vi "Funktionen Schalten Compact LP Paccar.vi"(8 "Fehler (Eingang)":errorcluster) -> (0 "Fehler (Ausgang)":errorcluster, 2 "Zustand":T1)   [LabVIEW 2020, in "Allgemein.lvlib"]
uses:
  Allgemein.lvlib
  Aktionen FGV Dichtheitstest.ctl
  FGV Zustaende Aktionen.ctl
  Verwaltung/Verwaltung - cRIO.lvlib
  Verwaltung/FGV OUT Aktionen.ctl
  Regler/Regler.lvlib
  Regler/FGV Daten Regler Aktionen.ctl
  Aktion FGV Messbetrieb.ctl
  Funktionstasten/Zustaende.ctl
  Funktionstasten/Funktionstasten.lvlib
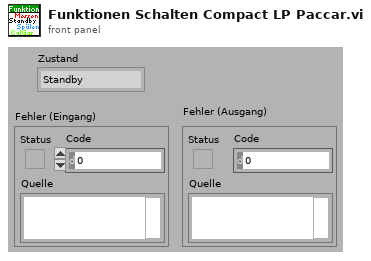
[diagram p1: front panel]
types:
  T1 = typedef "Funktionstasten.lvlib/Zustaende.ctl" = enum16{"Standby", "Pause", "Eco", "Messen", "Kalibrieren", "Spülen Filter", "Spülen Leitung", "Umgebungsluft", "0-Gas", "Cal-Gas", "CG zu PNS", "-------------", "Init 1", "Init 2", "Init 3", "Init 4", "Messen vorbereiten", "Messen durchführen", "Exit"}
  T2 = typedef "Allgemein.lvlib/Aktion FGV Messbetrieb.ctl" = enum16{"lesen", "schreiben"}
  T3 = typedef "Regler.lvlib/FGV Daten Regler Aktionen.ctl" = enum16{"lesen", "Out%", "Heizung EIN"}
  T4 = typedef "Verwaltung - cRIO.lvlib/FGV OUT Aktionen.ctl" = enum16{"lesen", "ANA OUT", "DO 0-31", "DO 32-47"}
  T5 = typedef "Allgemein.lvlib/FGV Zustaende Aktionen.ctl" = enum16{"lesen", "Zustand PC", "Zustand cRIO", "Bildnummer", "Samplepoint", "Sysloglevel"}
  T6 = typedef "Allgemein.lvlib/Aktionen FGV Dichtheitstest.ctl" = enum16{"lesen", "schreiben"}
  T7 = typedef "EPA 1065.lvlib/Dichtheitstest 1065-345.lvlib/Aktion Leak check durchfuehren.ctl" = enum16{"initialisieren", "Unterdruck erzeugen", "Ventile schließen", "Warten", "Auswertung", "fertig", "PDF erstellen"}
  T8 = typedef "Erweiterte Konfig.lvlib/Aktionen Dichtheitstest.ctl" = enum16{"Initialisieren", "Unterdruck aufbauen", "Prop schließen", "Warten", "Auswertung", "Fertig"}
  T9 = cluster{"-23Y1 (CG1)":bool, "-23Y2 (CG2)":bool, "-23Y3 (CG3-10)":bool, "-23Y4 (N2)":bool, "-23Y5":bool, "-27Y2":bool, "-20Y5":bool, "-20Y6":bool, "-20Y7":bool, "-20Y8":bool, "-27Y3":bool, "-27Y4":bool, "Pumpe":bool, "Kondensat":bool, "-22Y3":bool, "-20Y2":bool, "-21Y3":bool, "Absaugung":bool, "-21Y5":bool, "CG zu Entnahme":bool, "-20Y2 (CG3)":bool, "-20Y3 (CG4)":bool, "-20Y4 (CG5)":bool, "-20Y5 (CG6)":bool, "-20Y6 (CG7)":bool, "-20Y7 (CG8)":bool, "-20Y8 (CG9)":bool, "-21Y1 (CG10)":bool}
  T10 = typedef "Verwaltung - cRIO.lvlib/Digital Ausgaenge 32-63.ctl" = cluster{"O32: Messgaspumpe EIN":bool, "O33: (Umgebungsluftpumpe)":bool, "O34: (Kondensatpumpe GK)":bool, "O35: Klima/Lüfter EIN":bool, "O36: Versorgung Heizungen":bool, "O37: Versorgung Heizungen":bool, "O38: (Gaskühler EIN (Freigabe))":bool, "O39: Störung FAS LP":bool, "O40: (Heizung Filterblock)":bool, "O41: Heizung HL zu FT-IR":bool, "O42: Heizung HL Extern SP1":bool, "O43: Heizung HL Extern SP2":bool, "O44: Heizung Reserve":bool, "O45: Heizung Reserve":bool, "O46: Statusbeleuchtung grün":bool, "O47: Statusbeleuchtung rot":bool}
  T11 = typedef "Verwaltung - cRIO.lvlib/Digital Ausgaenge 0-31.ctl" = cluster{"O0: Druckluft Versorgung":bool, "O1: CG 3 (FB Eingang 1)":bool, "O2: CG 4 (Kühlung FT-IR EIN)":bool, "O3: CG 5 (FB Bypass)":bool, "O4: CG 6 (FB CalGas)":bool, "O5: CG 7 (FB spülen/UL)":bool, "O6: CG 8 (FB zum FT-IR)":bool, "O7: CG 9 (FB zum FID)":bool, "O8: CG 10 (FB Reserve)":bool, "O9: (FB Reserve)":bool, "O10: (FB Umgebungsluft FID)":bool, "O11: (FB zum Gaskühler)":bool, "O12: FB Stickstoff zu FT-IR":bool, "O13: (FB Druckluft/UL)":bool, "O14: (Purifier deaktivieren)":bool, "O15: (Umschaltung Purifier/Stickstoff)":bool, "O16: N2 Einblasung":bool, "O17: LSP LN2 Nachfüllung":bool, "O18: (Reserve)":bool, "O19: (Pumpe Eingang1)":bool, "O20: (Pumpe Eingang2)":bool, "O21: (Pumpe Spülen1)":bool, "O22: (Pumpe Spülen2)":bool, "O23: (Reserve)":bool, "O24: CalGas 1":bool, "O25: CalGas 2":bool, "O26: CG 3-10 (CalGas 3)":bool, "O27: Stickstoff aufschalten":bool, "O28: CG zu PNS":bool, "O29: FTIR Standby Spülung":bool, "O30: CG zu Entnahme(T90)":bool, "O31: (Purifier regenerieren)":bool}
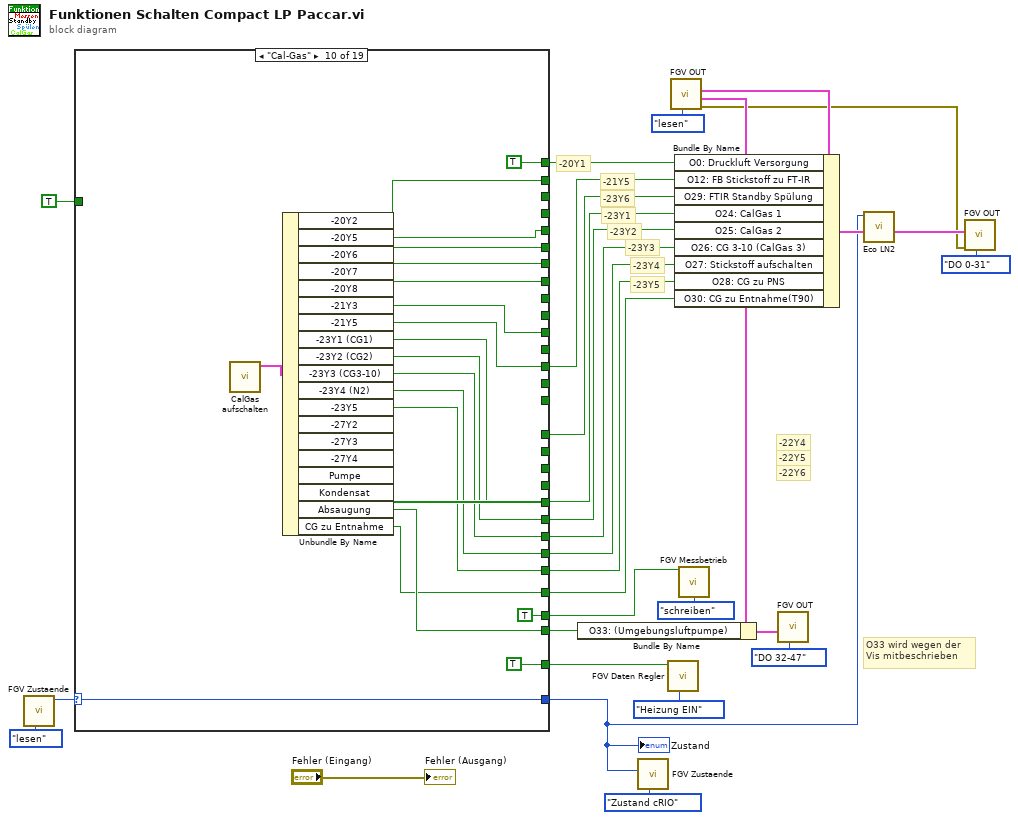
[diagram p0: block diagram]
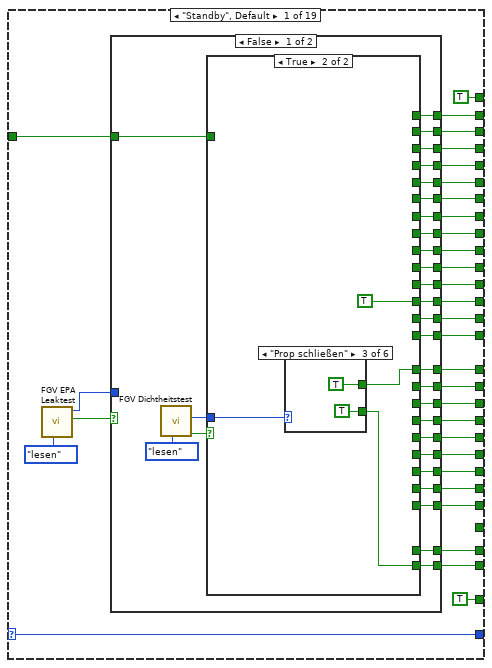
[diagram p2: hidden frame]
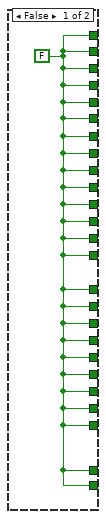
[diagram p3: hidden frame]
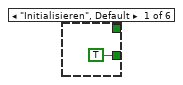
[diagram p4: hidden frame]
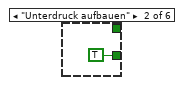
[diagram p5: hidden frame]
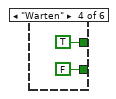
[diagram p6: hidden frame]
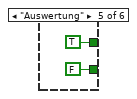
[diagram p7: hidden frame]
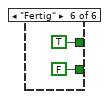
[diagram p8: hidden frame]
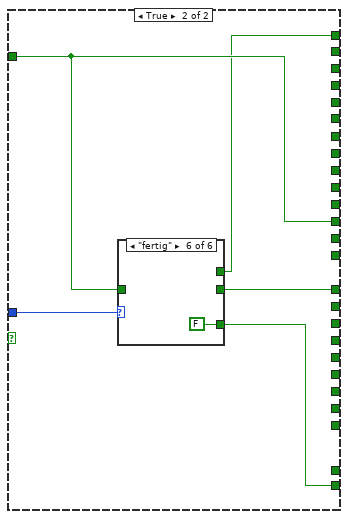
[diagram p9: hidden frame]
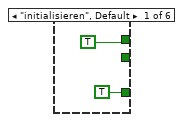
[diagram p10: hidden frame]
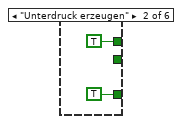
[diagram p11: hidden frame]
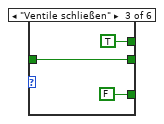
[diagram p12: hidden frame]
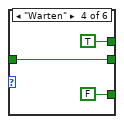
[diagram p13: hidden frame]
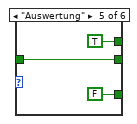
[diagram p14: hidden frame]
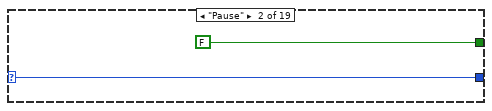
[diagram p15: hidden frame]
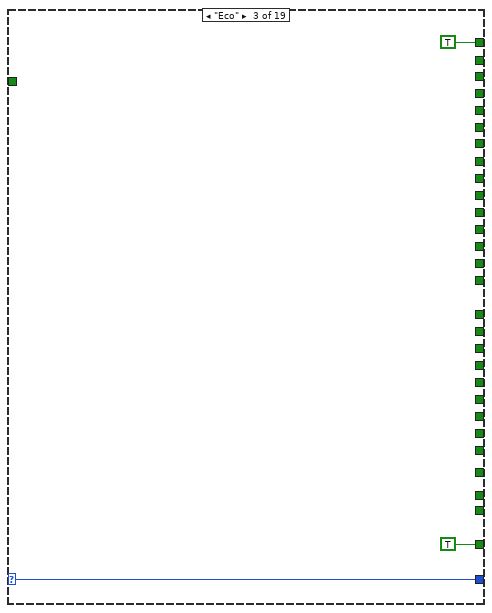
[diagram p16: hidden frame]
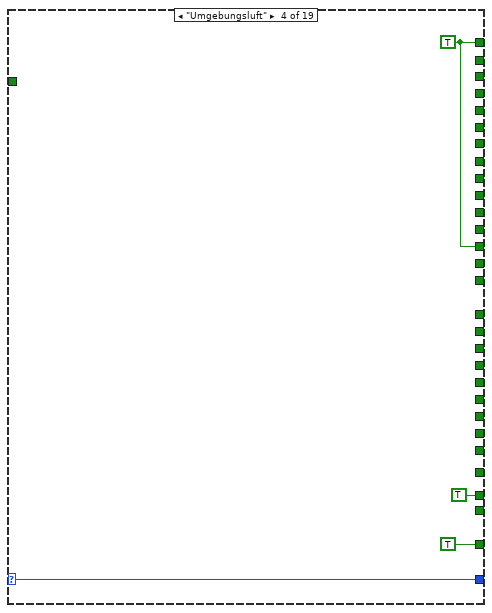
[diagram p17: hidden frame]
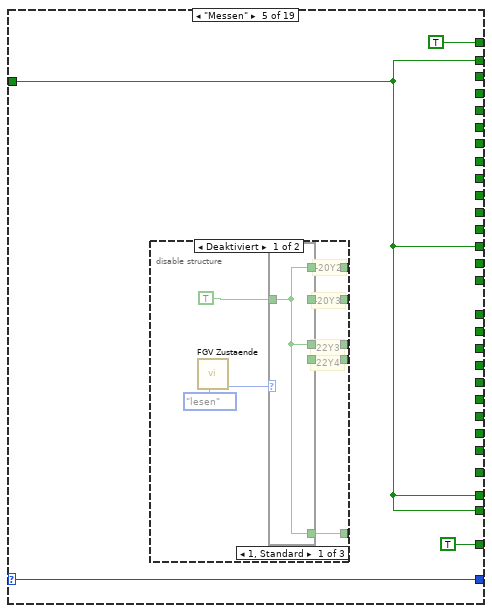
[diagram p18: hidden frame]
diagram:
  # "-23Y5"
  # "-23Y4"
  # "-23Y3"
  # "-23Y2"
  # "-23Y1"
  # "-23Y6"
  # "-21Y5"
  # "O33 wird wegen der \nVis mitbeschrieben"
  # "-20Y1"
  # "-22Y6"
  # "-22Y5"
  # "-22Y4"
  n1 = call "FGV Zustaende.vi"("Aktionen"=FGV_Zustaende_Aktionen."lesen") -> ("Zustand PC"=w20:T1)  [unwired: 6 in, 4 out]
  n2 = case shown="\"Cal-Gas\"" w20 {
    selector: w20 -> [w61 w126 w129 w133 w137 w179 w202 w206 w222 w241 w260 _ _ _ _ _ w262 w263 _]
    tunnel: [w61 w126 w129 w133 w137 w179 w202 w206 w222 w241 w260 _ _ _ _ _ w262 w263 _] -> w1
    tunnel: [w59 _ _ _ w134 w173 _ w203 _ w237 w256 _ _ _ _ _ _ _ _] -> _
    tunnel: [w58 _ _ _ _ w172 _ _ _ _ _ _ _ _ _ _ _ _ _] -> _
    tunnel: [w56 _ _ _ _ w170 _ _ w219 w236 w255 _ _ _ _ _ _ _ _] -> _
    tunnel: [w55 _ _ _ _ w169 _ _ _ w235 w254 _ _ _ _ _ _ _ _] -> _
    tunnel: [w54 _ _ _ _ w168 _ _ _ w234 w253 _ _ _ _ _ _ _ _] -> _
    tunnel: [w53 _ _ _ _ w167 _ _ _ w233 w252 _ _ _ _ _ _ _ _] -> _
    tunnel: [w52 _ _ _ _ w165 _ _ _ _ _ _ _ _ _ _ _ _ _] -> _
    tunnel: [w50 _ _ w131 w134 w162 _ _ w220 w231 w251 _ _ _ _ _ _ _ _] -> w27
    tunnel: [w49 _ _ _ _ w161 w199 w203 _ _ _ _ _ _ _ _ _ _ _] -> _
    tunnel: TRUE -> [w60 _ _ _ w134 _ w199 w203 w220 _ _ _ _ _ _ _ _ _ _]
    tunnel: [w57 _ _ _ _ w171 w198 _ _ _ _ _ _ _ _ _ _ _ _] -> _
    tunnel: [w48 _ _ _ _ w160 _ _ _ _ _ _ _ _ _ _ _ _ _] -> _
    tunnel: [w40 _ _ _ w134 w150 _ _ w220 w225 w246 _ _ _ _ _ _ _ _] -> w10
    tunnel: [w41 _ _ TRUE ("Pumpe") w134 w149 _ _ TRUE ("Pumpe") TRUE ("Pumpe") w245 _ _ _ _ _ _ _ _] -> w6
    tunnel: [w43 _ _ _ _ w155 _ _ _ w230 w250 _ _ _ _ _ _ _ _] -> w25
    tunnel: [w44 _ _ _ _ w156 _ _ _ _ _ _ _ _ _ _ _ _ _] -> _
    tunnel: [w45 _ _ _ _ w157 _ _ _ _ _ _ _ _ _ _ _ _ _] -> _
    tunnel: [w46 _ _ _ _ w158 _ _ _ _ _ _ _ _ _ _ _ _ _] -> _
    tunnel: [w47 _ _ _ _ w159 _ _ _ _ _ _ _ _ _ _ _ _ _] -> w26
    tunnel: [w42 _ _ _ _ w153 _ _ _ w228 w248 _ _ _ _ _ _ _ _] -> w24
    tunnel: [TRUE ("O0: Druckluft Versorgung") _ TRUE ("O0: Druckluft Versorgung") w131 TRUE ("O0: Druckluft Versorgung") TRUE ("O0: Druckluft Versorgung") TRUE ("O0: Druckluft Versorgung") TRUE ("O0: Druckluft Versorgung") w219 TRUE ("O0: Druckluft Versorgung") TRUE ("O0: Druckluft Versorgung") _ _ _ _ _ _ _ _] -> w28
    tunnel: [w38 _ _ _ _ w166 _ _ _ _ _ _ _ _ _ _ _ _ _] -> _
    tunnel: [w37 _ _ _ _ w163 _ _ _ _ _ _ _ _ _ _ _ _ _] -> _
    tunnel: [w36 _ _ _ _ w154 _ _ _ w229 w249 _ _ _ _ _ _ _ _] -> w8
    tunnel: [w35 _ _ _ _ w151 _ _ _ w226 w244 _ _ _ _ _ _ _ _] -> w23
    tunnel: [w34 _ _ _ _ w152 _ _ w220 w227 w247 _ _ _ _ _ _ _ _] -> w22
    tunnel: [TRUE ("Heizung AUS") FALSE ("Heizung AUS") TRUE ("Heizung AUS") TRUE ("Heizung AUS") TRUE ("Heizung AUS") TRUE ("Heizung AUS") TRUE ("Heizung AUS") TRUE ("Heizung AUS") TRUE ("Heizung AUS") TRUE ("Heizung AUS") TRUE ("Heizung AUS") TRUE ("Heizung AUS") _ _ _ _ _ _ _] -> w11
    tunnel: [w51 _ _ _ _ w164 _ _ _ w232 w243 _ _ _ _ _ _ _ _] -> _
    tunnel: [_ _ _ _ _ _ _ _ _ w223 w242 _ _ _ _ _ _ _ _] -> w5
    frame "Standby", Default {
      n3 = call "FGV EPA Leaktest.vi"("Aktion"=enum16{"lesen", "schreiben"}."lesen") -> ("Leaktest aktiv"=w31:bool, "Leaktest Zustand"=w30:T7)  [unwired: 9 in]
      n4 = case shown="False" w31 {
        tunnel: w60 -> [w90 w108]
        tunnel: [w89 w107] -> w59
        tunnel: [w88 _] -> w58
        tunnel: [w87 _] -> w57
        tunnel: [w86 _] -> w56
        tunnel: [w85 _] -> w55
        tunnel: [w84 _] -> w54
        tunnel: [w83 _] -> w53
        tunnel: [w82 _] -> w52
        tunnel: [w81 _] -> w51
        tunnel: [w80 w108] -> w50
        tunnel: [w79 _] -> w49
        tunnel: [w78 _] -> w48
        tunnel: [w77 w109] -> w47
        tunnel: [w76 _] -> w46
        tunnel: [w75 _] -> w45
        tunnel: [w74 _] -> w44
        tunnel: [w73 _] -> w43
        tunnel: [w72 _] -> w42
        tunnel: [w71 _] -> w41
        tunnel: [w70 w106] -> w40
        tunnel: [w67 _] -> w38
        tunnel: [w66 _] -> w37
        tunnel: [w65 _] -> w36
        tunnel: [w64 _] -> w35
        tunnel: [w63 _] -> w34
        tunnel: w30 -> [_ w110]
        frame False {
          n5 = call "FGV Dichtheitstest.vi"("Aktionen"=Aktionen_FGV_Dichtheitstest."lesen") -> ("Dichtheitstest?"=w68:bool, "Aktionen Dichtheitstest"=w62:T8)  [unwired: 9 in]
          n6 = case shown="True" w68 {
            tunnel: [w91 _] -> w89
            tunnel: [w91 w92] -> w70
            tunnel: [w91 _] -> w71
            tunnel: [w91 _] -> w72
            tunnel: [w91 _] -> w73
            tunnel: [w91 _] -> w74
            tunnel: [w91 _] -> w75
            tunnel: [w91 _] -> w76
            tunnel: [w91 w93] -> w77
            tunnel: [w91 _] -> w78
            tunnel: [w91 _] -> w79
            tunnel: [w91 TRUE] -> w80
            tunnel: [w91 _] -> w81
            tunnel: [w91 _] -> w82
            tunnel: [w91 _] -> w83
            tunnel: [w91 _] -> w84
            tunnel: [w91 _] -> w85
            tunnel: [w91 _] -> w86
            tunnel: [w91 _] -> w87
            tunnel: [w91 _] -> w88
            tunnel: w90 -> [_ _]
            tunnel: [w91 _] -> w67
            tunnel: [w91 _] -> w66
            tunnel: [w91 _] -> w65
            tunnel: [w91 _] -> w64
            tunnel: [w91 _] -> w63
            tunnel: w62 -> [_ w94]
            frame False {
              w91 = FALSE
            }
            frame True {
              n7 = case shown="\"Prop schließen\"" w94 {
                tunnel: [_ _ TRUE TRUE TRUE TRUE] -> w93
                tunnel: [TRUE TRUE TRUE FALSE FALSE FALSE] -> w92
                frame "Initialisieren", Default {
                }
                frame "Unterdruck aufbauen" {
                }
                frame "Prop schließen" {
                }
                frame "Warten" {
                }
                frame "Auswertung" {
                }
                frame "Fertig" {
                }
              }
            }
          }
        }
        frame True {
          n8 = case shown="\"fertig\"" w110 {
            tunnel: w108 -> [_ _ w117 w120 w123 _]
            tunnel: [_ _ w117 w120 w123 _] -> w109
            tunnel: [TRUE TRUE TRUE TRUE TRUE _] -> w107
            tunnel: [TRUE TRUE FALSE FALSE FALSE FALSE] -> w106
            frame "initialisieren", Default {
            }
            frame "Unterdruck erzeugen" {
            }
            frame "Ventile schließen" {
            }
            frame "Warten" {
            }
            frame "Auswertung" {
            }
            frame "fertig" {
            }
          }
        }
      }
    }
    frame "Pause" {
    }
    frame "Eco" {
    }
    frame "Umgebungsluft" {
      w131 = TRUE ("O0: Druckluft Versorgung")
    }
    frame "Messen" {
      n9 = disable-structure shown="Deaktiviert" {
        disable-tunnel: [w145 _] -> _
        disable-tunnel: [w144 _] -> _
        disable-tunnel: [w143 _] -> _
        disable-tunnel: [w142 _] -> _
        disable-tunnel: [w141 _] -> _
        frame Disabled {
          # "-22Y4"
          # "-22Y3"
          # "-20Y2"
          # "-20Y3"
          n10 = call "FGV Zustaende.vi"("Aktionen"=FGV_Zustaende_Aktionen."lesen") -> ("Samplepoint"=w138:u16)  [unwired: 6 in, 4 out]
          n11 = case shown="1, Standard" w138 {
            tunnel: TRUE -> [w146 w147 w148]
            tunnel: [w146 _ _] -> w145
            tunnel: [w146 w147 _] -> w144
            tunnel: [_ w147 _] -> w143
            tunnel: [_ _ w148] -> w142
            tunnel: [w146 w147 _] -> w141
            frame 1, Default {
            }
            frame 2 {
            }
            frame 3 {
            }
          }
        }
        frame Enabled {
        }
      }
    }
    frame "Kalibrieren" {
      n12 = call "FGV Dichtheitstest.vi"("Aktionen"=Aktionen_FGV_Dichtheitstest."lesen") -> ("Dichtheitstest?"=w175:bool, "Aktionen Dichtheitstest"=w174:T8)  [unwired: 9 in]
      n13 = case shown="True" w175 {
        tunnel: [w182 _] -> w173
        tunnel: [w182 w183] -> w150
        tunnel: [w181 _] -> w149
        tunnel: [w182 _] -> w153
        tunnel: [w182 _] -> w155
        tunnel: [w182 _] -> w156
        tunnel: [w182 _] -> w157
        tunnel: [w182 _] -> w158
        tunnel: [w182 w184] -> w159
        tunnel: [w182 _] -> w160
        tunnel: [w182 _] -> w161
        tunnel: [TRUE TRUE] -> w162
        tunnel: [w182 _] -> w164
        tunnel: [w182 _] -> w165
        tunnel: [w182 _] -> w167
        tunnel: [w182 _] -> w168
        tunnel: [w182 _] -> w169
        tunnel: [w182 _] -> w170
        tunnel: [w182 _] -> w171
        tunnel: [w182 _] -> w172
        tunnel: [w182 _] -> w166
        tunnel: [w182 _] -> w163
        tunnel: [w182 _] -> w154
        tunnel: [w181 _] -> w151
        tunnel: [w181 _] -> w152
        tunnel: w174 -> [_ w185]
        frame False {
          w181 = TRUE
          w182 = FALSE
        }
        frame True {
          n14 = case shown="\"Warten\"" w185 {
            tunnel: [_ _ TRUE TRUE TRUE TRUE] -> w184
            tunnel: [TRUE TRUE TRUE FALSE FALSE FALSE] -> w183
            frame "Initialisieren", Default {
            }
            frame "Unterdruck aufbauen" {
            }
            frame "Prop schließen" {
            }
            frame "Warten" {
            }
            frame "Auswertung" {
            }
            frame "Fertig" {
            }
          }
        }
      }
    }
    frame "Spülen Filter" {
      n15 = call "Taktmerker.vi"("Aktion"=enum16{"lesen", "bearbeiten"}."lesen") -> ("1 s"=w198:bool)  [unwired: 6 in, 4 out]
    }
    frame "Spülen Leitung" {
      n16 = disable-structure shown="Deaktiviert" {
        disable-tunnel: [w214 _] -> _
        disable-tunnel: [w213 _] -> _
        disable-tunnel: [w212 _] -> _
        disable-tunnel: [w211 _] -> _
        disable-tunnel: [w210 _] -> _
        frame Disabled {
          # "-22Y6"
          # "-22Y5"
          # "-21Y7"
          # "-20Y6"
          # "-20Y3"
          n17 = call "FGV Zustaende.vi"("Aktionen"=FGV_Zustaende_Aktionen."lesen") -> ("Samplepoint"=w207:u16)  [unwired: 6 in, 4 out]
          n18 = case shown="3" w207 {
            tunnel: TRUE -> [w215 w216 w217]
            tunnel: [w215 _ _] -> w214
            tunnel: [_ w216 _] -> w213
            tunnel: [_ _ w217] -> w212
            tunnel: [_ _ w217] -> w211
            tunnel: [_ _ w217] -> w210
            frame 1, Default {
            }
            frame 2 {
            }
            frame 3 {
            }
          }
        }
        frame Enabled {
        }
      }
    }
    frame "0-Gas" {
      w219 = TRUE ("O0: Druckluft Versorgung")
    }
    frame "Cal-Gas" {
      n19 = call "CalGas aufschalten.vi"() -> ("Cluster"=w238:T9)  [unwired: 11 in]
      n20 = Unbundle By Name(w238) -> ("-20Y2"=w237:bool, "-20Y5"=w236:bool, "-20Y6"=w235:bool, "-20Y7"=w234:bool, "-20Y8"=w233:bool, "-21Y3"=w232:bool, "-21Y5"=w231:bool, "-23Y1 (CG1)"=w230:bool, "-23Y2 (CG2)"=w229:bool, "-23Y3 (CG3-10)"=w228:bool, "-23Y4 (N2)"=w227:bool, "-23Y5"=w226:bool, "Absaugung"=w225:bool, "CG zu Entnahme"=w223:bool)  [unwired: 5 out]
    }
    frame "CG zu PNS" {
      n21 = call "CalGas aufschalten.vi"() -> ("Cluster"=w257:T9)  [unwired: 11 in]
      n22 = Unbundle By Name(w257) -> ("-20Y2"=w256:bool, "-20Y5"=w255:bool, "-20Y6"=w254:bool, "-20Y7"=w253:bool, "-20Y8"=w252:bool, "-21Y3"=w243:bool, "-21Y5"=w251:bool, "-23Y1 (CG1)"=w250:bool, "-23Y2 (CG2)"=w249:bool, "-23Y3 (CG3-10)"=w248:bool, "-23Y4 (N2)"=w247:bool, "-23Y5"=w244:bool, "Pumpe"=w245:bool, "Absaugung"=w246:bool, "CG zu Entnahme"=w242:bool)  [unwired: 4 out]
    }
    frame "-------------" {
    }
    frame "Init 1" {
    }
    frame "Init 2" {
    }
    frame "Init 3" {
    }
    frame "Init 4" {
    }
    frame "Messen vorbereiten" {
    }
    frame "Messen durchführen" {
    }
    frame "Exit" {
    }
  }
  "Zustand" <- w1
  n23 = call "FGV Zustaende.vi"("Aktionen"=FGV_Zustaende_Aktionen."Zustand cRIO", "Zustand cRIO"=w1) -> ()  [unwired: 5 in, 5 out]
  n24 = call "FGV Daten Regler.vi"("Aktionen"=FGV_Daten_Regler_Aktionen."Heizung EIN", "Heizung EIN"=w11) -> ()  [unwired: 8 in, 2 out]
  n25 = call "FGV OUT.vi"("Aktion"=FGV_OUT_Aktionen."lesen") -> ("error out"=w2:errorcluster, "DO 32-63"=w16:T10, "DO 0-31"=w17:T11)  [unwired: 7 in, 1 out]
  n26 = Bundle By Name(cluster=w16, "O33: (Umgebungsluftpumpe)"=w10) -> (w13:T10)
  n27 = Bundle By Name(cluster=w17, "O0: Druckluft Versorgung"=w28, "O12: FB Stickstoff zu FT-IR"=w27, "O29: FTIR Standby Spülung"=w26, "O24: CalGas 1"=w25, "O25: CalGas 2"=w8, "O26: CG 3-10 (CalGas 3)"=w24, "O27: Stickstoff aufschalten"=w22, "O28: CG zu PNS"=w23, "O30: CG zu Entnahme(T90)"=w5) -> (w4:T11)
  n28 = call "FGV Messbetrieb.vi"("messen"=w6, "Aktion"=Aktion_FGV_Messbetrieb."schreiben") -> ()  [unwired: 12 in, 2 out]
  n29 = call "FGV OUT.vi"("Aktion"=FGV_OUT_Aktionen."DO 32-47", "DO 32-63"=w13) -> ()  [unwired: 6 in, 4 out]
  n30 = call "Eco LN2.vi"("DO 0-31"=w4, "Zustand cRIO"=w1) -> ("DO 0-31 2"=w3:T11)  [unwired: 8 in, 1 out]
  n31 = call "FGV OUT.vi"("Aktion"=FGV_OUT_Aktionen."DO 0-31", "error in (no error)"=w2, "DO 0-31"=w3) -> ()  [unwired: 5 in, 4 out]
  "Fehler (Ausgang)" <- "Fehler (Eingang)"
